vi "DAQmx Write (Digital 1D Bool 1Chan 1Samp).vi"(0 "task/channels in":refnum<k21>, 1 "auto start":bool=TRUE, 7 "data":bool[](array[boolean]), 9 "timeout":dbl=10.0 format="%0.2f", 11 "error in":errorcluster) -> (4 "task out":refnum<k21>, 10 "number of samples written per channel":u32, 15 "error out":errorcluster)   [LabVIEW 2022 SP3]
doc: "Writes a single sample of Boolean values to a task that contains a single digital output channel. The channel can contain one or more digital lines."
uses:
  nilvaiu.dll
panel:
  # "line"
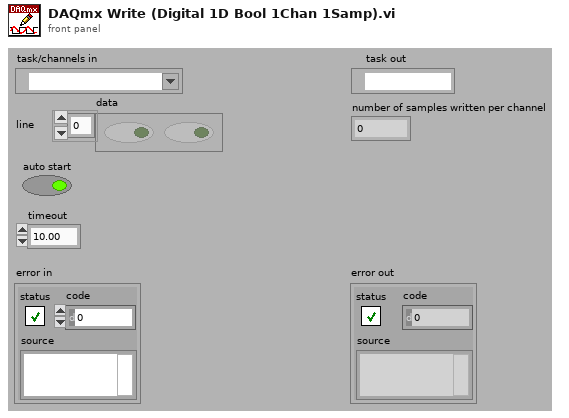
[diagram p1: front panel]
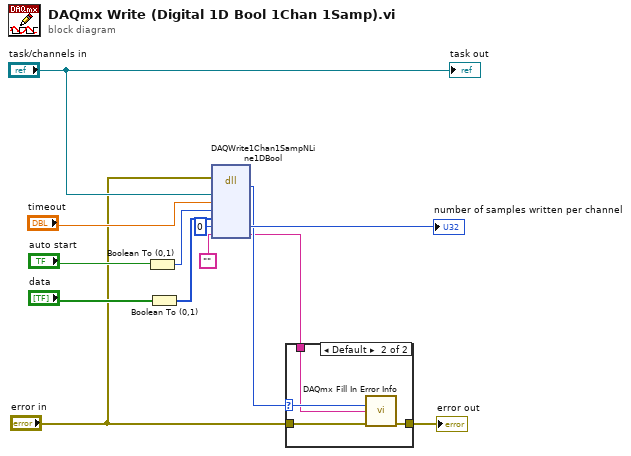
[diagram p0: block diagram]
diagram:
  n1 = Boolean To (0,1)(Boolean="auto start") -> (0, 1=w5:i16)
  n2 = Boolean To (0,1)(Boolean="data") -> (0, 1=w2:i16[])
  n3 = dll-call lib="nilvaiu.*" fn="DAQWrite1Chan1SampNLine1DBool"(error in="error in", "taskID"="task/channels in", "timeout"="timeout", "autoStart"=w5, "data"=w2, "numSamplesWriten"=u32 0, "extendedErrorInfo"="") -> (w7:i32, "numSamplesWriten"=→"number of samples written per channel":u32, "extendedErrorInfo"=w4:string)  [unwired: 3 in, 5 out]
  n4 = case shown="Default" w7 {
    selector: w7 -> [_ w16]
    tunnel: "error in" -> [w14 w18]
    tunnel: [w14 w17] -> w12
    tunnel: w4 -> [_ w15]
    frame 0 {
    }
    frame Default {
      n5 = call "DAQmx Fill In Error Info.vi"("status code"=w16, "extended error info"=w15, "error in"=w18) -> ("error out"=w17:errorcluster)  [unwired: 1 in, 11 out]
    }
  }
  "error out" <- w12
  "task out" <- "task/channels in"
